vi "Zustände schalten.vi"(7 "Samplepoint setzen":bool, 8 "error in (no error)":errorcluster caption="Fehler (Eingang, kein Fehler)", 9 "Samplepoint 2":string, 10 "T90":bool, 11 "Zustand":T1) -> (0 "error out":errorcluster caption="Fehler (Ausgang)")   [LabVIEW 2020, in "Amium PNS.lvlib"]
uses:
  Amium PNS.lvlib
  Funktionstasten/Zustaende.ctl
  Aktion FGV Amium Daten.ctl
  Seiten/Erweiterte Konfig/FGV PID Aktionen.ctl
  AK Kommunikation/Amium Kommandos verwalten Aktionen.ctl
  Seiten/CalGas Aufschaltung/FGV CalGas Aktionen.ctl
  AK Kommunikation/AK Kommunikation.lvlib
  Seiten/CalGas Aufschaltung/CalGas Aufschaltung.lvlib
  Seiten/Erweiterte Konfig/Erweiterte Konfig.lvlib
  Funktionstasten/Funktionstasten.lvlib
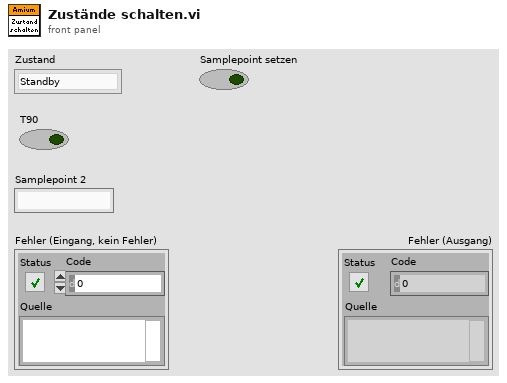
[diagram p1: front panel]
types:
  T1 = typedef "Funktionstasten.lvlib/Zustaende.ctl" = enum16{"Standby", "Pause", "Eco", "Messen", "Kalibrieren", "Spülen Filter", "Spülen Leitung", "Umgebungsluft", "0-Gas", "Cal-Gas", "CG zu PNS", "-------------", "Init 1", "Init 2", "Init 3", "Init 4", "Messen vorbereiten", "Messen durchführen", "Exit"}
  T2 = typedef "Amium PNS.lvlib/Aktion FGV Amium Daten.ctl" = enum16{"lesen", "Komm Daten", "Daten", "Error", "Regler", "Grenzwerte", "laden", "speichern"}
  T3 = typedef "Erweiterte Konfig.lvlib/FGV PID Aktionen.ctl" = enum16{"Lesen", "Schreiben PID", "Schreiben Sonstige", "Dichtheitstest", "Aktionen Dicht.", "Parameter Sensor"}
  T4 = typedef "Amium PNS.lvlib/AK Kommunikation.lvlib/Amium Kommandos verwalten Aktionen.ctl" = enum16{"lesen", "setzen Ende", "setzen Pos1", "senden", "initalisieren", "prüfen", "Kommandos"}
  T5 = typedef "CalGas Aufschaltung.lvlib/FGV CalGas Aktionen.ctl" = enum16{"lesen", "Analysator Auswahl", "Def.CalGas", "Aufschaltung CalGas", "laden", "speichern", "KAL extrahieren"}
  T6 = typedef "Amium PNS.lvlib/Daten Cluster.ctl" = cluster{"Amium Zustände":T7, "Samplepoint am PNS":i16, "Gerätekennung":string, "aktiver Samplepoint":i16[], "Messgasdruck":sgl}
  T7 = typedef "Amium PNS.lvlib/Amium Zustand.ctl" = u16
  T8 = typedef "CalGas Aufschaltung.lvlib/Aufschaltung CalGas.ctl" = cluster{"Kalibriergas":T9, "Aufschaltpunkt":T10, "Analysator":T11}
  T9 = typedef "Auswahlfeld.ctl" = u16
  T10 = typedef "CalGas Aufschaltung.lvlib/Auswahl Aufschaltpunkt.ctl" = enum16{"über Filterblock", "Analysator direkt", "über PNS", "Entnahme", "Gasdivider"}
  T11 = typedef "CalGas Aufschaltung.lvlib/Auswahl Analysator.ctl" = enum16{"FT-IR", "FID", "PMA", "PMA/FID/FT-IR"}
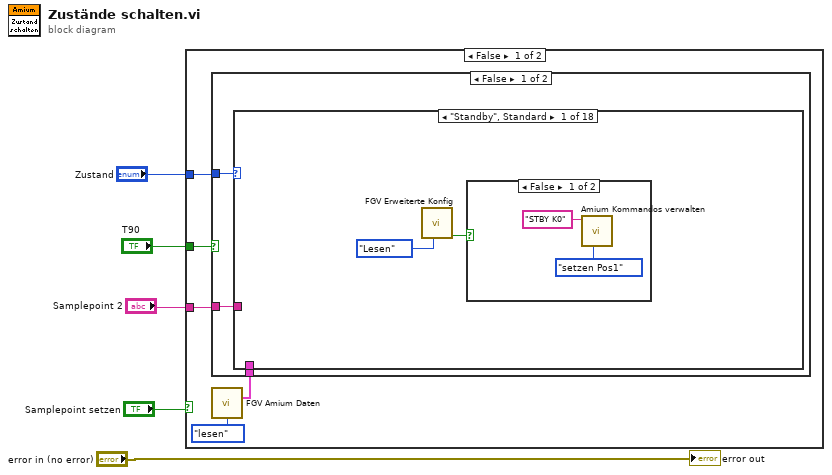
[diagram p0: block diagram]
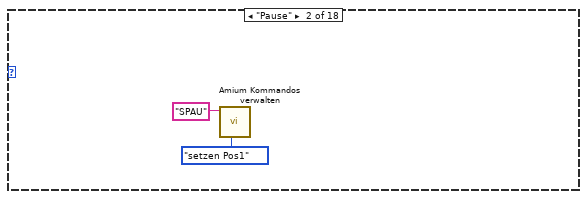
[diagram p3: hidden frame]
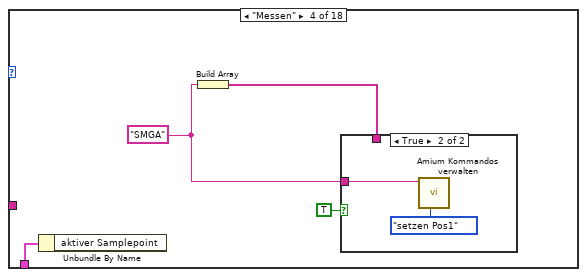
[diagram p5: hidden frame]
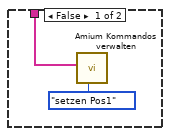
[diagram p6: hidden frame]
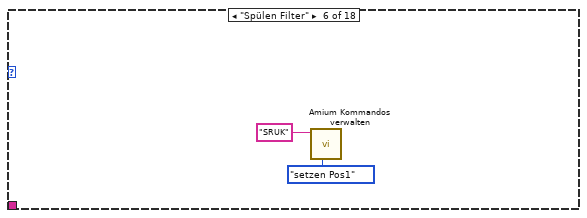
[diagram p8: hidden frame]
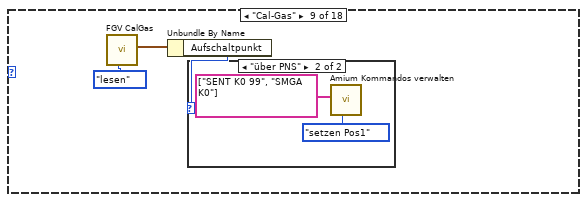
[diagram p11: hidden frame]
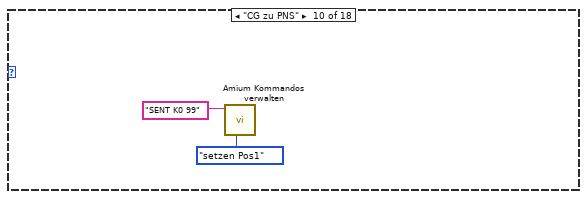
[diagram p13: hidden frame]
diagram:
  n1 = case shown="False" "Samplepoint setzen" {
    tunnel: "Zustand" -> [w10 _]
    tunnel: "Samplepoint 2" -> [w9 w37]
    tunnel: "T90" -> [w8 _]
    frame False {
      n2 = call "FGV Amium Daten.vi"("Aktion"=Aktion_FGV_Amium_Daten."lesen") -> ("Amium Daten"=w6:T6)  [unwired: 9 in, 5 out]
      n3 = case shown="False" w8 {
        tunnel: w10 -> [w13 _]
        tunnel: w9 -> [w12 _]
        tunnel: w6 -> [w11 _]
        frame False {
          n4 = case shown="\"Standby\", Standard" w13 {
            tunnel: w12 -> [_ _ _ _ _ _ _ _ _ _ _ _ _ _ _ _ _ _]
            tunnel: w11 -> [_ _ _ w23 _ _ _ _ _ _ _ _ _ _ _ _ _ _]
            frame "Standby", Default {
              n5 = call "FGV Erweiterte Konfig.vi"("Aktion"=FGV_PID_Aktionen."Lesen") -> ("Dichtheitstest?"=w15:bool)  [unwired: 6 in, 4 out]
              n6 = case shown="False" w15 {
                frame False {
                  n7 = call "Amium Kommandos verwalten.vi"("Aktionen"=Amium_Kommandos_verwalten_Aktionen."setzen Pos1", "neues Kommando"="STBY K0") -> ()  [unwired: 7 in, 3 out]
                }
                frame True {
                }
              }
            }
            frame "Pause" {
              n8 = call "Amium Kommandos verwalten.vi"("Aktionen"=Amium_Kommandos_verwalten_Aktionen."setzen Pos1", "neues Kommando"="SPAU") -> ()  [unwired: 7 in, 3 out]
            }
            frame "Eco" {
            }
            frame "Messen" {
              w21 = "SMGA"
              n9 = Unbundle By Name(w23) -> ()  [unwired: 1 out]
              n10 = Build Array(w21) -> (w22:string[])
              n11 = case shown="True" TRUE {
                tunnel: w22 -> [w24 _]
                tunnel: w21 -> [_ w26]
                frame False {
                  n12 = call "Amium Kommandos verwalten.vi"("Aktionen"=Amium_Kommandos_verwalten_Aktionen."setzen Pos1", "neues Kommando Array"=w24) -> ()  [unwired: 7 in, 3 out]
                }
                frame True {
                  n13 = call "Amium Kommandos verwalten.vi"("Aktionen"=Amium_Kommandos_verwalten_Aktionen."setzen Pos1", "neues Kommando"=w26) -> ()  [unwired: 7 in, 3 out]
                }
              }
            }
            frame "Kalibrieren" {
            }
            frame "Spülen Filter" {
              # "#PNStakten"
              n14 = call "Amium Kommandos verwalten.vi"("Aktionen"=Amium_Kommandos_verwalten_Aktionen."setzen Pos1", "neues Kommando"="SRUK") -> ()  [unwired: 7 in, 3 out]
            }
            frame "Spülen Leitung" {
            }
            frame "0-Gas" {
            }
            frame "Cal-Gas" {
              n15 = call "FGV CalGas.vi"("Aktionen"=FGV_CalGas_Aktionen."lesen") -> ("Aufschaltung CalGas"=w31:T8)  [unwired: 6 in, 4 out]
              n16 = Unbundle By Name(w31) -> ("Aufschaltpunkt"=w30:T10)
              n17 = case shown="\"über PNS\"" w30 {
                frame "über Filterblock", Default {
                }
                frame "über PNS" {
                  n18 = call "Amium Kommandos verwalten.vi"("Aktionen"=Amium_Kommandos_verwalten_Aktionen."setzen Pos1", "neues Kommando Array"=string[] ["SENT K0 99", "SMGA K0"]) -> ()  [unwired: 7 in, 3 out]
                }
              }
            }
            frame "CG zu PNS" {
              n19 = call "Amium Kommandos verwalten.vi"("Aktionen"=Amium_Kommandos_verwalten_Aktionen."setzen Pos1", "neues Kommando"="SENT K0 99") -> ()  [unwired: 7 in, 3 out]
            }
            frame "-------------" {
            }
            frame "Init 1" {
            }
            frame "Init 2" {
            }
            frame "Init 3" {
            }
            frame "Init 4" {
            }
            frame "Messen vorbereiten" {
            }
            frame "Messen durchführen" {
            }
            frame "Exit" {
            }
          }
        }
        frame True {
          # "#T90LP"
        }
      }
    }
    frame True {
      n20 = Concatenate Strings("SENT K0", w37) -> (w38:string)
      n21 = call "Amium Kommandos verwalten.vi"("Aktionen"=Amium_Kommandos_verwalten_Aktionen."setzen Pos1", "neues Kommando"=w38) -> ()  [unwired: 7 in, 3 out]
    }
  }
  "error out" <- "error in (no error)"
